vi "set_frekans_array.vi"(10 "LstBox Refnum":refnum<vi>) -> (2 "Array":dbl[](array[numeric]))   [LabVIEW 2014]
panel:
  out "size(s)":i32
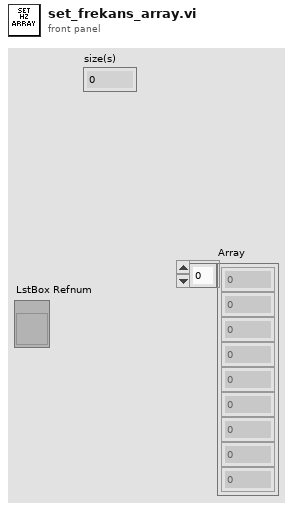
[diagram p1: front panel]
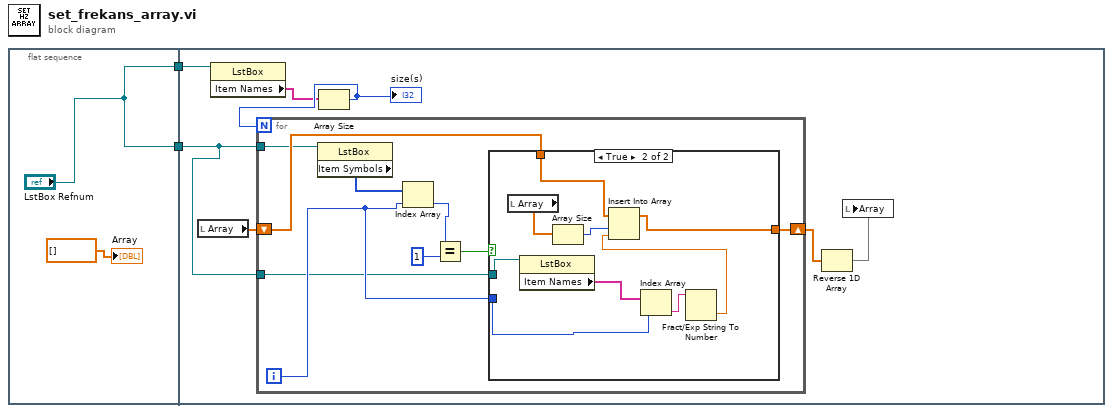
[diagram p0: block diagram]
diagram:
  n1 = flat-sequence {
    tunnel: ["LstBox Refnum"] -> w2
    tunnel: ["LstBox Refnum"] -> w1
    tunnel: w2 -> [w7]
    tunnel: w1 -> [w6]
    frame #0 {
      "Array" <- dbl[] [] ("Array")
    }
    frame #1 {
      n2 = local read "Array"() -> (w9:dbl[])
      n3 = property class="LstBox"(reference=w7) -> ("Item Names"=w5:string[])  [unwired: 1 in, 2 out]
      n4 = Array Size(array=w5) -> (size(s)=w8:i32)
      "size(s)" <- w8
      n5 = for {
        N: w8 -> [_]
        shift-right: [w16] -> w10
        shift-left: w9 -> [w17]
        tunnel: w6 -> [w13]
        tunnel: w6 -> [w12]
        i -> [w15]
        n6 = property class="LstBox"(reference=w13) -> ("Item Symbols"=w14:i32[])  [unwired: 1 in, 2 out]
        n7 = Index Array(array=w14, index=w15) -> (element=w20:i32)
        n8 = Equal?(x=w20, y=1) -> (x = y?=w18:bool)
        n9 = case shown="True" w18 {
          tunnel: w17 -> [w21 w30]
          tunnel: [w21 w27] -> w16
          tunnel: w15 -> [_ w26]
          tunnel: w12 -> [_ w22]
          frame False {
          }
          frame True {
            n10 = local read "Array"() -> (w25:dbl[])
            n11 = property class="LstBox"(reference=w22) -> ("Item Names"=w23:string[])  [unwired: 1 in, 2 out]
            n12 = Array Size(array=w25) -> (size(s)=w24:i32)
            n13 = Index Array(array=w23, index=w26) -> (element=w29:string)
            n14 = Fract/Exp String To Number(string=w29) -> (number=w28:dbl)  [unwired: 3 in, 1 out]
            n15 = Insert Into Array(array=w30, index=w24, new element=w28) -> (w27:dbl[])
          }
        }
      }
      n16 = Reverse 1D Array(array=w10) -> (reversed array=w11:dbl[])
      n17 = local write "Array"(w11) -> ()
    }
  }
